vi "ScopeInstrument_CallCreateSessionWithUnregisteredSessionReserved_RemoteSessionCreated.vi"(8 "error in":errorcluster) -> (0 "error out":errorcluster, 2 "result":string, 3 "pass":bool)   [LabVIEW 2020, in "MeasurementServerTests.lvlib"]
uses:
  MeasurementServerTests.lvlib
  Runtime/MeasurementLink Session Management/Session Reservation/Session Reservation.lvclass
  Runtime/MeasurementLink niScope/Create Sessions - 1Sess.vi
  Runtime/MeasurementLink niScope/MeasurementLink niScope.lvlib
panel:
  out "session reservation out":refnum<class "Session Reservation.lvclass">
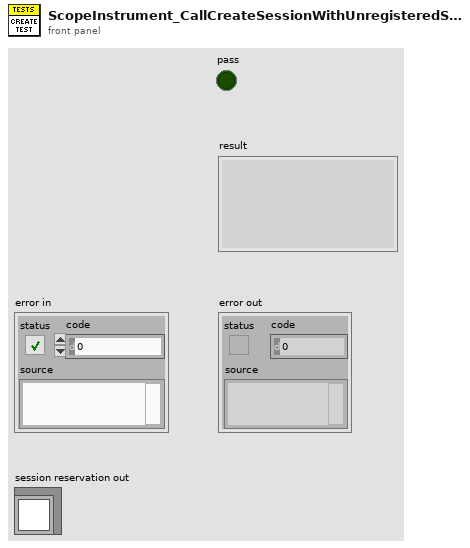
[diagram p1: front panel]
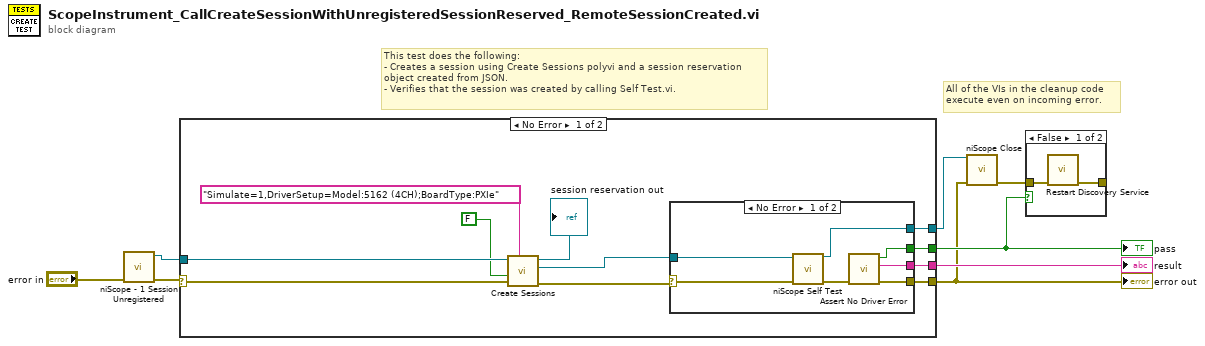
[diagram p0: block diagram]
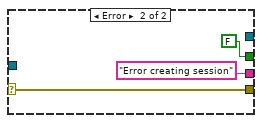
[diagram p2: hidden frame]
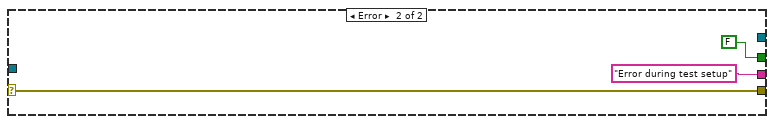
[diagram p3: hidden frame]
diagram:
  # "All of the VIs in the cleanup code\nexecute even on incoming error."
  # "This test does the following:\n- Creates a session using Create Sessions polyvi and a session reservation\nobject created from JSON.\n- Verifies that the session was created by calling Self Test.vi."
  n1 = call "niScope - 1 Session Unregistered.vi"("error in"="error in") -> ("error out"=w2:errorcluster, "Session Reservation out"=w1:refnum<class "Session Reservation.lvclass">)  [unwired: 9 in]
  n2 = case shown="No Error" w2 {
    selector: w2 -> [w12 w30]
    tunnel: [w18 w30] -> w4
    tunnel: [w19 FALSE] -> w5
    tunnel: [w17 "Error during test setup" ("f")] -> w8
    tunnel: [w16 _] -> w7
    tunnel: w1 -> [w11 _]
    frame No Error {
      n3 = call-poly "Create Sessions.vi"("option string"="Simulate=1,DriverSetup=Model:5162 (4CH);BoardType:PXIe", "error in"=w12, "reset"=FALSE, "session reservation in"=w11) -> ("error out"=w10:errorcluster, "session"=w13:refnum<k15>, "session reservation out"=→"session reservation out":refnum<class "Session Reservation.lvclass">)  [unwired: 4 in, 1 out]
      n4 = case shown="No Error" w10 {
        selector: w10 -> [w20 w28]
        tunnel: [w26 FALSE] -> w19
        tunnel: [w24 w28] -> w18
        tunnel: [w25 "Error creating session"] -> w17
        tunnel: w13 -> [w21 _]
        tunnel: [w23 _] -> w16
        frame No Error {
          n5 = call <instrlib>:"niScope Self Test.vi"("instrument handle"=w21, "error in"=w20) -> ("instrument handle out"=w23:refnum<k15>, "error out"=w22:errorcluster)  [unwired: 10 in, 2 out]
          n6 = call "Assert No Driver Error.vi"("error in"=w22) -> ("error out"=w24:errorcluster, "result"=w25:string, "pass?"=w26:bool)  [unwired: 8 in]
        }
        frame Error {
        }
      }
    }
    frame Error {
    }
  }
  "error out" <- w4
  "pass" <- w5
  "result" <- w8
  n7 = call <instrlib>:"niScope Close.vi"("instrument handle"=w7, "error in"=w4) -> ("error out"=w6:errorcluster)  [unwired: 13 in]
  n8 = case shown="False" w5 {
    tunnel: w6 -> [w34 _]
    tunnel: [w33 _] -> _
    frame False {
      n9 = call "Restart Discovery Service.vi"("error in"=w34) -> ("error out"=w33:errorcluster)  [unwired: 10 in]
    }
    frame True {
    }
  }
